vi "GDX_Chart.vi"() -> ()   [LabVIEW 2019]
panel:
  out "Waveform Chart":dbl[][](graph)
  in  "stop":bool
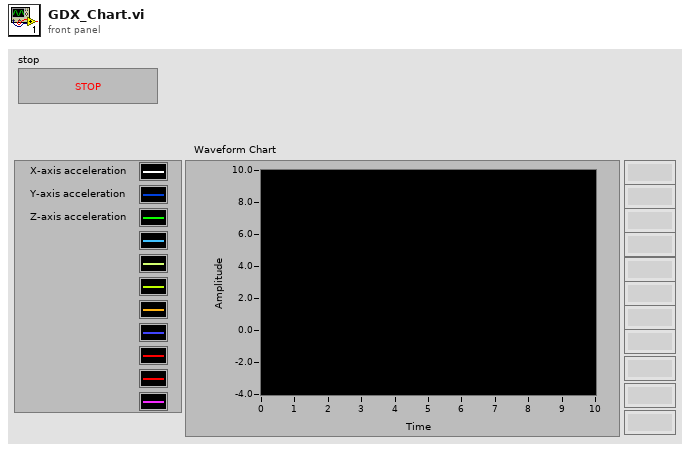
[diagram p1: front panel]
types:
  T1 = enum16{"Activate from Dialog Popup", "Activate All Channels", "Input On/Off Array", "Input Channel  Mask", "Burn Sensor Default Channels"}
  T2 = enum16{"Set Rate from Dialog Popup", "Default 1 Sample/Sec", "Input Sample Rate"}
  T3 = typedef "D2PIO_D2PIOCluster.ctl" = cluster{"Library Handle":i64, "Device List Handle":i64, "BT Device Handles":i64[], "USB Device Handles":i64[], "BT+USB Device Handles":i64[], "Measurement Tick":dbl[], "Ch Availability Mask":u32[]}
  T4 = typedef "D2PIO_ChannelInfoCluster.ctl" = cluster{"Channel":i8, "Ch is Active":bool, "Channel ID":u32, "Channel Description":string, "Channel Unit":string}[]
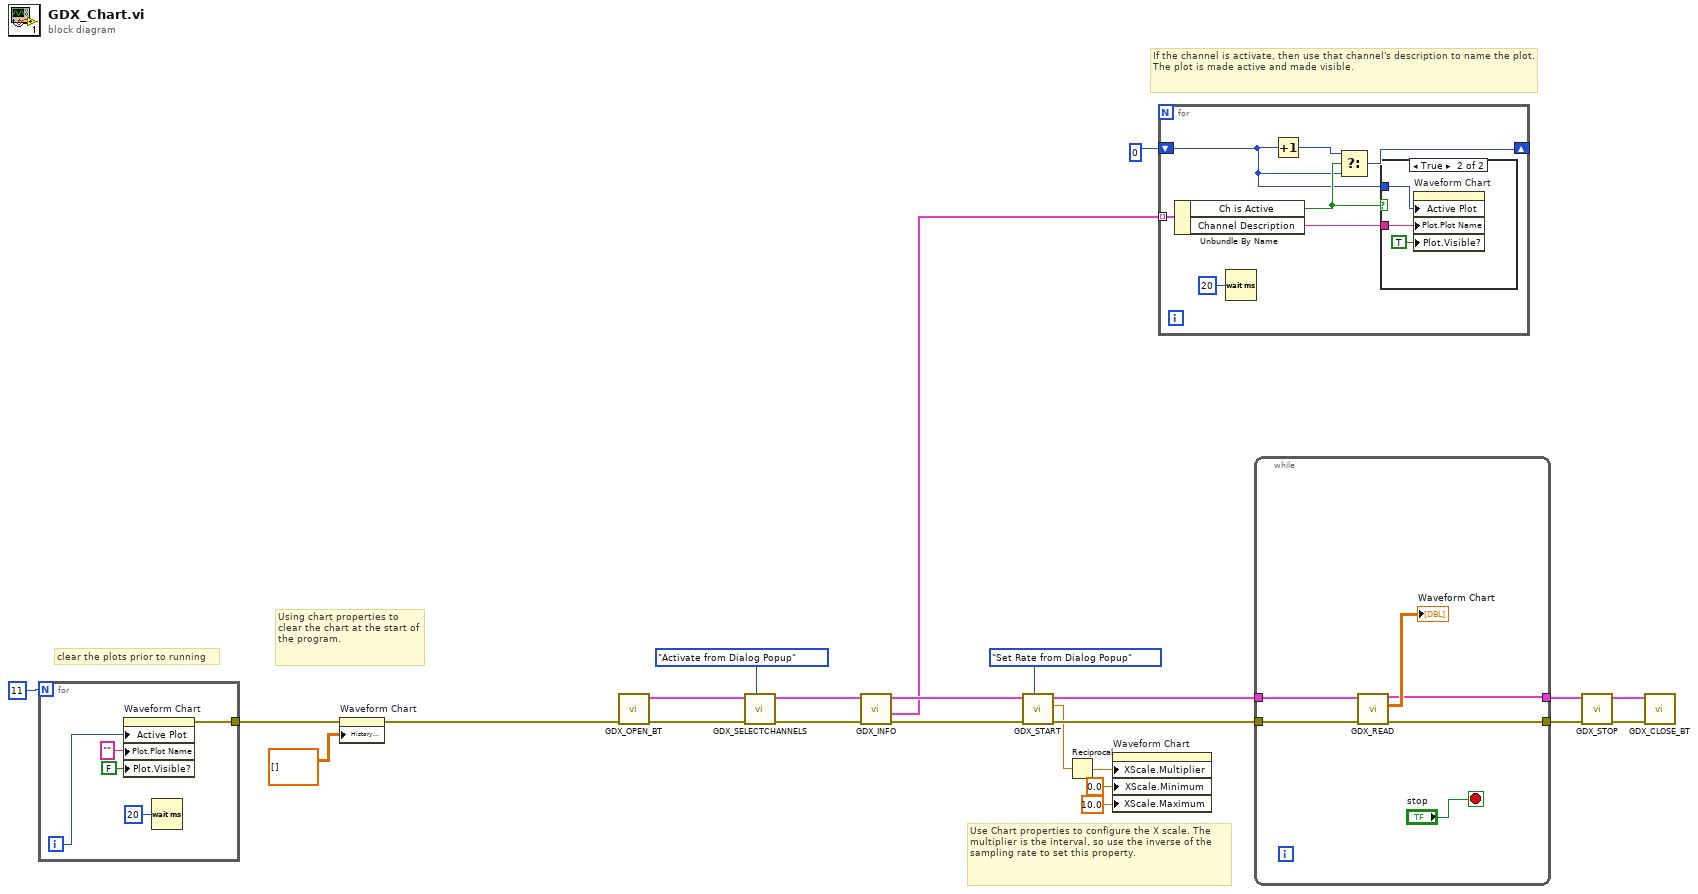
[diagram p0: block diagram]
diagram:
  # "If the channel is activate, then use that channel's description to name the plot. The plot is made active and made visible."
  # "clear the plots prior to running"
  # "Use Chart properties to configure the X scale. The multiplier is the interval, so use the inverse of the sampling rate to set this property."
  # "Using chart properties to clear the chart at the start of the program."
  n1 = for {
    N: 11 -> [_]
    tunnel: [w25] -> w7
    i -> [w27]
    n2 = property on="Waveform Chart" class="WFChart (strict)"("Active Plot"=w27, "Plot.Plot Name"="", "Plot.Visible?"=FALSE ("Plot.Visible")) -> (error out=w25:errorcluster)  [unwired: 2 in, 1 out]
    n3 = Wait (ms)(milliseconds to wait=u32 20) -> ()  [unwired: 1 out]
  }
  n4 = property on="Waveform Chart" class="WFChart (strict)"(error in=w7, "History Data"=dbl[][] []) -> (error out=w9:errorcluster)  [unwired: 1 in, 1 out]
  n5 = call <vilib>:"GDX_OPEN_BT.vi"("error in (no error)"=w9) -> ("error out"=w18:errorcluster, "D2PIO Cluster Out"=w19:T3)  [unwired: 9 in]
  n6 = call <vilib>:"GDX_SELECTCHANNELS.vi"("Enum"=T1."Activate from Dialog Popup", "error in (no error)"=w18, "D2PIO Cluster In"=w19) -> ("error out"=w4:errorcluster, "D2PIO Cluster Out"=w5:T3)  [unwired: 7 in]
  n7 = call <vilib>:"GDX_INFO.vi"("error in (no error)"=w4, "D2PIO Cluster In"=w5) -> ("error out"=w3:errorcluster, "Array of Channel Info Cluster"=w1:T4, "D2PIO Cluster Out"=w2:T3)  [unwired: 4 in, 3 out]
  n8 = call <vilib>:"GDX_START.vi"("Enum"=T2."Set Rate from Dialog Popup", "error in (no error)"=w3, "D2PIO Cluster In"=w2) -> ("error out"=w24:errorcluster, "Actual Sample Rate"=w16:dbl, "D2PIO Cluster Out"=w23:T3)  [unwired: 5 in, 1 out]
  n9 = Reciprocal(x=w16) -> (1/x=w15:dbl)
  n10 = property on="Waveform Chart" class="WFChart (strict)"("XScale.Multiplier"=w15, "XScale.Minimum"=0.0 ("X Scale.Range:Minimum"), "XScale.Maximum"=10.0 ("X Scale.Range:Maximum")) -> ()  [unwired: 2 in, 2 out]
  n11 = for {
    tunnel: w1 -> [w36] mode=indexing
    shift-right: [w32] -> _
    shift-left: u32 0 ("Active Plot") -> [w30]
    n12 = Unbundle By Name(w36) -> ("Ch is Active"=w33:bool, "Channel Description"=w35:string)
    n13 = Wait (ms)(milliseconds to wait=u32 20) -> ()  [unwired: 1 out]
    n14 = Increment(x=w30) -> (x+1=w31:u32)
    n15 = Select(t=w31, s=w33, f=w30) -> (s? t:f=w32:u32)
    n16 = case shown="True" w33 {
      tunnel: w35 -> [_ w39]
      tunnel: w30 -> [_ w38]
      frame False {
      }
      frame True {
        n17 = property on="Waveform Chart" class="WFChart (strict)"("Active Plot"=w38, "Plot.Plot Name"=w39, "Plot.Visible?"=TRUE ("Plot.Visible")) -> ()  [unwired: 2 in, 2 out]
      }
    }
  }
  n18 = while {
    tunnel: w24 -> [w45]
    tunnel: w23 -> [w43]
    tunnel: [w40] -> w22
    tunnel: [w41] -> w17
    stop <- "stop" stop-if-true
    n19 = call <vilib>:"GDX_READ.vi"("error in (no error)"=w45, "D2PIO Cluster In"=w43) -> ("error out"=w41:errorcluster, "Waveform Chart Data"=→"Waveform Chart":dbl[][], "D2PIO Cluster Out"=w40:T3)  [unwired: 4 in, 3 out]
  }
  n20 = call <vilib>:"GDX_STOP.vi"("error in (no error)"=w17, "D2PIO Cluster In"=w22) -> ("error out"=w20:errorcluster, "D2PIO Cluster Out"=w21:T3)  [unwired: 8 in]
  n21 = call <vilib>:"GDX_CLOSE_BT.vi"("error in (no error)"=w20, "D2PIO Cluster In"=w21) -> ()  [unwired: 8 in, 2 out]
